vi "Get Groups.vi"(8 "error in (no error)":errorcluster, 11 "ParseSVG in":refnum<class "ParseSVG.lvclass">) -> (0 "error out":errorcluster, 3 "ParseSVG out":refnum<class "ParseSVG.lvclass">)   [LabVIEW 2019, in "ParseSVG.lvclass"]
uses:
  ParseSVG.lvclass
  ParseSVG.lvclass/ParseSVG.ctl
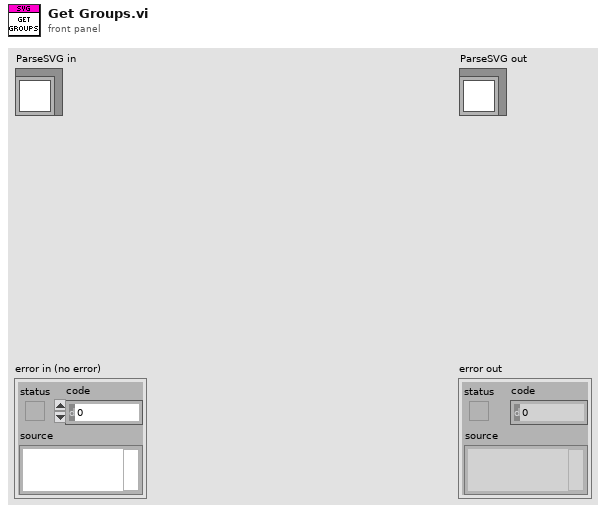
[diagram p1: front panel]
types:
  T1 = cluster{"Start":i32, "id":string, "transforms":string, "End":i32}[]
  T2 = cluster{i32, "RawXML":string, "RawXML":string, i32}[]
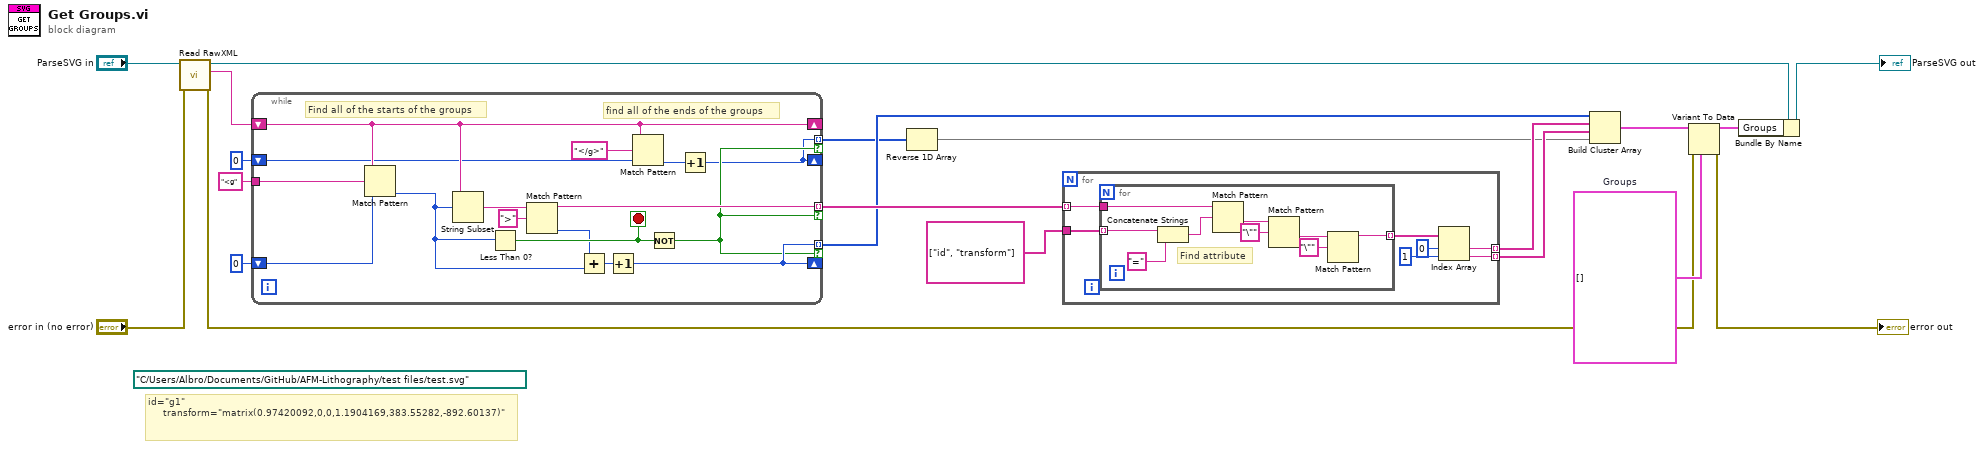
[diagram p0: block diagram]
diagram:
  (unwired) path "C:/Users/Albro/Documents/GitHub/AFM-Lithography/test files/test.svg" ("file (use dialog)")
  w9 = T1 []  # Groups
  # "id=\"g1\"\n     transform=\"matrix(0.97420092,0,0,1.1904169,383.55282,-892.60137)\""
  n1 = call "Read RawXML.vi"("error in (no error)"="error in (no error)", "ParseXML in"="ParseSVG in") -> ("error out"=w2:errorcluster, "RawXML"=w4:string, "ParseXML out"=w7:refnum<class "ParseSVG.lvclass">)  [unwired: 7 in]
  n2 = while {
    shift-right: [w29] -> _
    shift-left: w4 -> [w29]
    shift-right: [w26] -> _
    shift-left: 0 -> [w35]
    tunnel: [w32] -> w16 mode=indexing if=w25
    tunnel: "<g" -> [w21]
    tunnel: [w22] -> w11 mode=indexing if=w25
    tunnel: [w26] -> w12 mode=indexing if=w25
    shift-right: [w22] -> _
    shift-left: 0 ("offset past match") -> [w24]
    stop <- w31 stop-if-true
    # "Find all of the starts of the groups"
    # "find all of the ends of the groups"
    n3 = Match Pattern(string=w29, regular expression=w21, offset (0)=w35) -> (offset past match=w27:i32)  [unwired: 3 out]
    n4 = String Subset(string=w29, offset (0)=w27) -> (substring=w36:string)  [unwired: 1 in]
    n5 = Less Than 0?(x=w27) -> (x < 0?=w31:bool)
    n6 = Match Pattern(string=w36, regular expression=">") -> (before substring=w32:string, offset past match=w30:i32)  [unwired: 1 in, 2 out]
    n7 = Add(x=w30, y=w27) -> (x+y=w34:i32)
    n8 = Increment(x=w34) -> (x+1=w26:i32)
    n9 = Match Pattern(string=w29, regular expression="</g>", offset (0)=w24) -> (offset past match=w23:i32)  [unwired: 3 out]
    n10 = Not(x=w31) -> (.not. x?=w25:bool)
    n11 = Increment(x=w23) -> (x+1=w22:i32)
  }
  n12 = Reverse 1D Array(array=w11) -> (reversed array=w1:i32[])
  n13 = for {
    tunnel: w16 -> [w43] mode=indexing
    tunnel: string[] ["id", "transform"] -> [w42]
    tunnel: [w38] -> w14 mode=indexing
    tunnel: [w37] -> w13 mode=indexing
    n14 = for {
      tunnel: w43 -> [w52]
      tunnel: w42 -> [w45] mode=indexing
      tunnel: [w44] -> w41 mode=indexing
      # "Find attribute"
      n15 = Concatenate Strings(w45, "=" ("string")) -> (w47:string)
      n16 = Match Pattern(string=w52, regular expression=w47) -> (after substring=w51:string)  [unwired: 1 in, 3 out]
      n17 = Match Pattern(string=w51, regular expression="\"") -> (after substring=w49:string)  [unwired: 1 in, 3 out]
      n18 = Match Pattern(string=w49, regular expression="\"") -> (before substring=w44:string)  [unwired: 1 in, 3 out]
    }
    n19 = Index Array(array=w41, index #1=0 ("index"), index #2=1 ("index")) -> (element #1=w38:string, element #2=w37:string)
  }
  n20 = Build Cluster Array(w12, w14, w13, w1) -> (w10:T2)
  n21 = Variant To Data(error in=w2, type=w9, Variant=w10) -> (data=w5:T1, error out=→"error out":errorcluster)
  n22 = Bundle By Name(cluster=w7, "Groups"=w5) -> (→"ParseSVG out":refnum<class "ParseSVG.lvclass">)
